vi "Status_FGV.vi"() -> ()   [LabVIEW 2011]
uses:
  Status_com.ctl
panel:
  out "State out":bool
  in  "State in":bool
  in  "command":T1
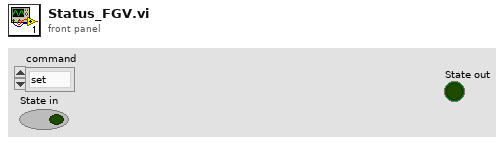
[diagram p1: front panel]
types:
  T1 = typedef "Status_com.ctl" = enum16{"set", "get", "init"}
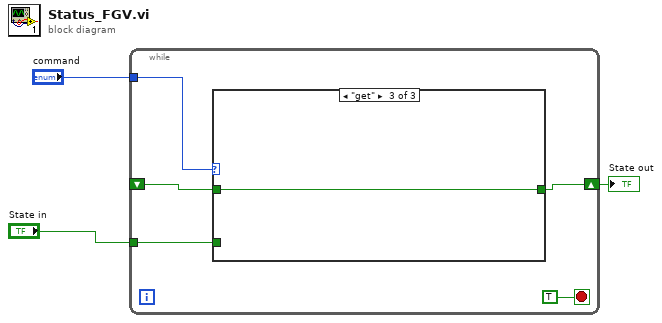
[diagram p0: block diagram]
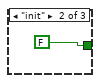
[diagram p3: hidden frame]
diagram:
  n1 = while {
    shift-right: [w7] -> w1
    shift-left: _ -> [w8]
    tunnel: "command" -> [w6]
    tunnel: "State in" -> [w5]
    stop <- TRUE stop-if-true
    n2 = case shown="\"get\"" w6 {
      tunnel: w8 -> [_ _ w11]
      tunnel: [w9 FALSE ("Boolean 2") w11] -> w7
      tunnel: w5 -> [w9 _ _]
      frame "set", Default {
      }
      frame "init" {
      }
      frame "get" {
      }
    }
  }
  "State out" <- w1
